vi "GT Buf Set Var Value.vi"(5 "fifo":i16, 6 "value":dbl, 7 "pVarInfo":T1, 8 "error in (no error)":errorcluster caption="错误输入（无错误）", 9 "pageId":i16, 10 "crd":i16, 11 "cardNum":i16) -> (0 "error out":errorcluster caption="错误输出", 2 "function return":i16, 3 "pVarInfo out":T1)   [LabVIEW 2014, in "gts.lvlib"]
doc: "GT_API GT_BufSetVarValue(short cardNum,short crd,short pageId,TVarInfo *pVarInfo,double value,short fifo=0);"
uses:
  gts.lvlib
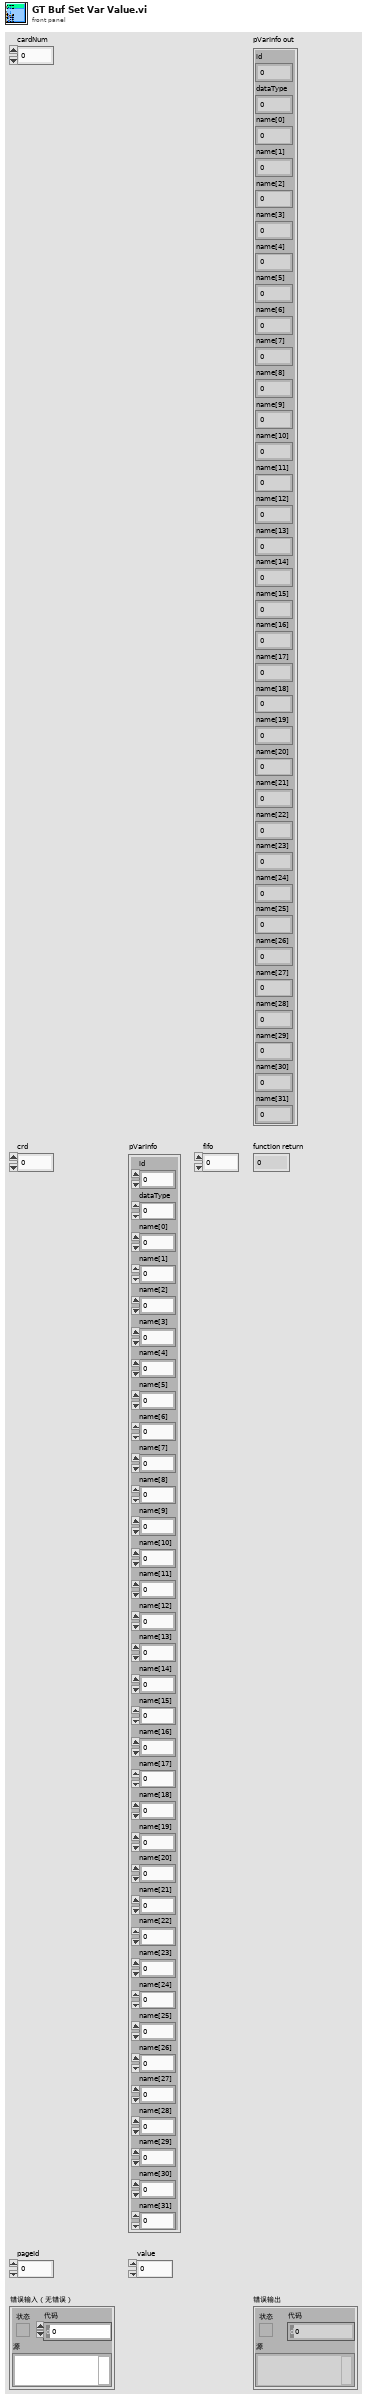
[diagram p1: front panel]
types:
  T1 = cluster{"id":i16, "dataType":i16, "name[0]":i8, "name[1]":i8, "name[2]":i8, "name[3]":i8, "name[4]":i8, "name[5]":i8, "name[6]":i8, "name[7]":i8, "name[8]":i8, "name[9]":i8, "name[10]":i8, "name[11]":i8, "name[12]":i8, "name[13]":i8, "name[14]":i8, "name[15]":i8, "name[16]":i8, "name[17]":i8, "name[18]":i8, "name[19]":i8, "name[20]":i8, "name[21]":i8, "name[22]":i8, "name[23]":i8, "name[24]":i8, "name[25]":i8, "name[26]":i8, "name[27]":i8, "name[28]":i8, "name[29]":i8, "name[30]":i8, "name[31]":i8}
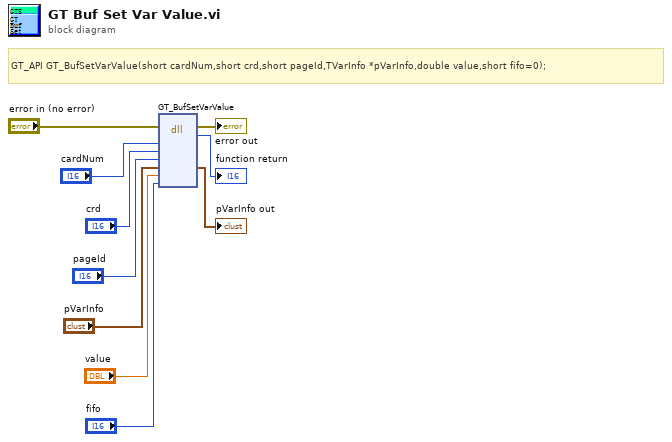
[diagram p0: block diagram]
diagram:
  # "GT_API GT_BufSetVarValue(short cardNum,short crd,short pageId,TVarInfo *pVarInfo,double value,short fifo=0);"
  n1 = dll-call lib="PTH2habs D固高科技资料GTS控制卡GTS卡18年上半年资料dllVC32bit\nmulti_cardgts.*" fn="GT_BufSetVarValue"(error in="error in (no error)", "cardNum"="cardNum", "crd"="crd", "pageId"="pageId", "pVarInfo"="pVarInfo", "value"="value", "fifo"="fifo") -> (error out=→"error out":errorcluster, →"function return":i16, "pVarInfo"=→"pVarInfo out":T1)  [unwired: 7 in, 1 out]
